vi "emi_Loop Control.vi"   [LabVIEW 2011]
doc: "Enable and disable loops by index(s)"
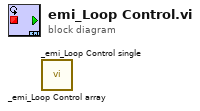
[diagram p0: block diagram]
diagram:
  n1 = call "_emi_Loop Control array.vi"() -> ()  [unwired: 14 in, 2 out]
  n2 = call "_emi_Loop Control single.vi"() -> ()  [unwired: 14 in, 2 out]
